vi "3.2.vi"() -> ()   [LabVIEW 2017]
panel:
  out "结果":dbl
  in  "B":dbl
  in  "A":dbl
  in  "枚举":enum16{"除", "乘", "减", "加"}(ring)
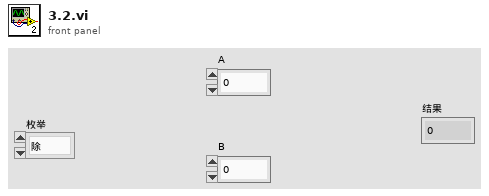
[diagram p1: front panel]
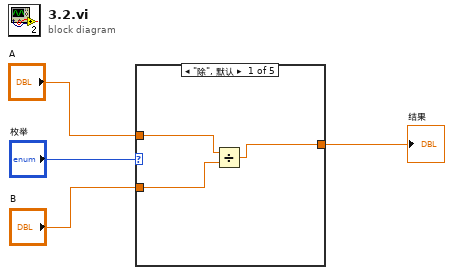
[diagram p0: block diagram]
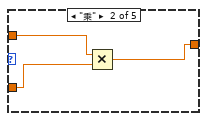
[diagram p2: hidden frame]
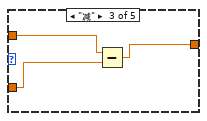
[diagram p3: hidden frame]
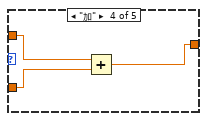
[diagram p4: hidden frame]
diagram:
  n1 = case shown="\"除\", 默认" "枚举" {
    tunnel: "A" -> [w7 w10 w13 w16 _]
    tunnel: "B" -> [w6 w9 w12 w15 _]
    tunnel: [w5 w8 w11 w14 _] -> w1
    frame "除", Default {
      n2 = Divide(x=w7, y=w6) -> (x/y=w5:dbl)
    }
    frame "乘" {
      n3 = Multiply(x=w10, y=w9) -> (x*y=w8:dbl)
    }
    frame "减" {
      n4 = Subtract(x=w13, y=w12) -> (x-y=w11:dbl)
    }
    frame "加" {
      n5 = Add(x=w16, y=w15) -> (x+y=w14:dbl)
    }
    frame ? {
    }
  }
  "结果" <- w1
